vi "RT test - Copy.vi"() -> ()   [LabVIEW 2014]
uses:
  <vilib>/Platform/TimedLoop/XDataNode/timing_clust.ctl
  <vilib>/Platform/TimedLoop/XDataNode/nitl_modes.ctl
  <vilib>/Platform/TimedLoop/XDataNode/wakeup.ctl
  <vilib>/FPGAPlugInAG/cRIO-9066/niLvFpga_Open_cRIO-9066.vi
  <vilib>/rvi/interface/common/dynamic/niFpgaDynamicAddResources.vi
  <vilib>/Utility/error.llb/Error Cluster From Error Code.vi
  <vilib>/rvi/errors/niLvFpgaAdjustHostInterfaceError.vi
  <vilib>/platform/TimedLoop/XDataNode/XDataNode.xnode
  <vilib>/rvi/interface/nirviOpenFPGA/nirviOpenFPGA.xnode
  FPGA Bitfiles/SMSLDrill_FPGATarget_SMSL-DrillFPGA_76AJMwWUk6w.lvbitx
  FPGA/SMSL-Drill FPGA.vi
  <vilib>/rvi/interface/nirviReadWriteControl/nirviReadWriteControl.xnode
  <vilib>/Platform/TimedLoop/XDataNode/XDNodeRunTimeDep.lvlib
  NiFpgaLv.dll
  <vilib>/rvi/interface/Simulation/niFpgaSimulationCallBeginRW.vi
  <vilib>/NI_Real-Time Target Support.lvlib
panel:
  in  "Enable/Disable":bool
  in  "Speed Command [Inch/S]":dbl
  in  "Inch / Step":dbl=0.1
  in  "Manual":bool
  in  "Frequency [Hz]":dbl
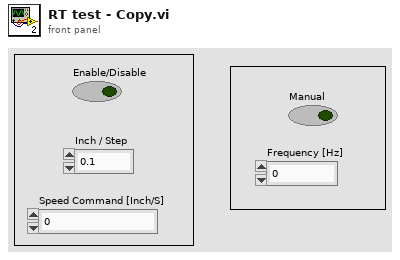
[diagram p1: front panel]
types:
  T1 = typedef "XDNodeRunTimeDep.lvlib/timing_clust.ctl" = cluster{"Expected End [f-1]":u64, "Actual End [f-1]":u64, "Finished Late? [f-1]":bool, "Expected End [i-1]":u64, "Actual End [i-1]":u64, "Finished Late? [i-1]":bool, "Expected Start [i]":u64, "Actual Start [i]":u64, "Expected Start [f]":u64, "Actual Start [f]":u64, "Source Name":string, "Structure Name":string, "Period":i64, "Deadline":i64, "Offset":i64, "Start":i64, "Priority":i32, "Timeout":i32, "Mode":T2, "Wakeup Reason":T3, "Error":errorcluster, "Source Type":string, "Secondary Source Type":string, "Global End Time":u64, "Global Start Time":u64, "Frame Duration":u64, "Iteration Duration":u64, "Assigned CPU":i32, "I/O Scan Engine Mode":u32}
  T2 = typedef "XDNodeRunTimeDep.lvlib/nitl_modes.ctl" = enum32{"No Change", "Process missed periods, maintain original phase", "Discard missed periods, maintain original phase", "Process missed periods, ignore original phase", "Discard missed periods, ignore original phase"}
  T3 = typedef "XDNodeRunTimeDep.lvlib/wakeup.ctl" = enum32{"Normal", "Aborted", "Asynchronous wakeup", "Timing source error", "Timed loop error", "Timeout"}
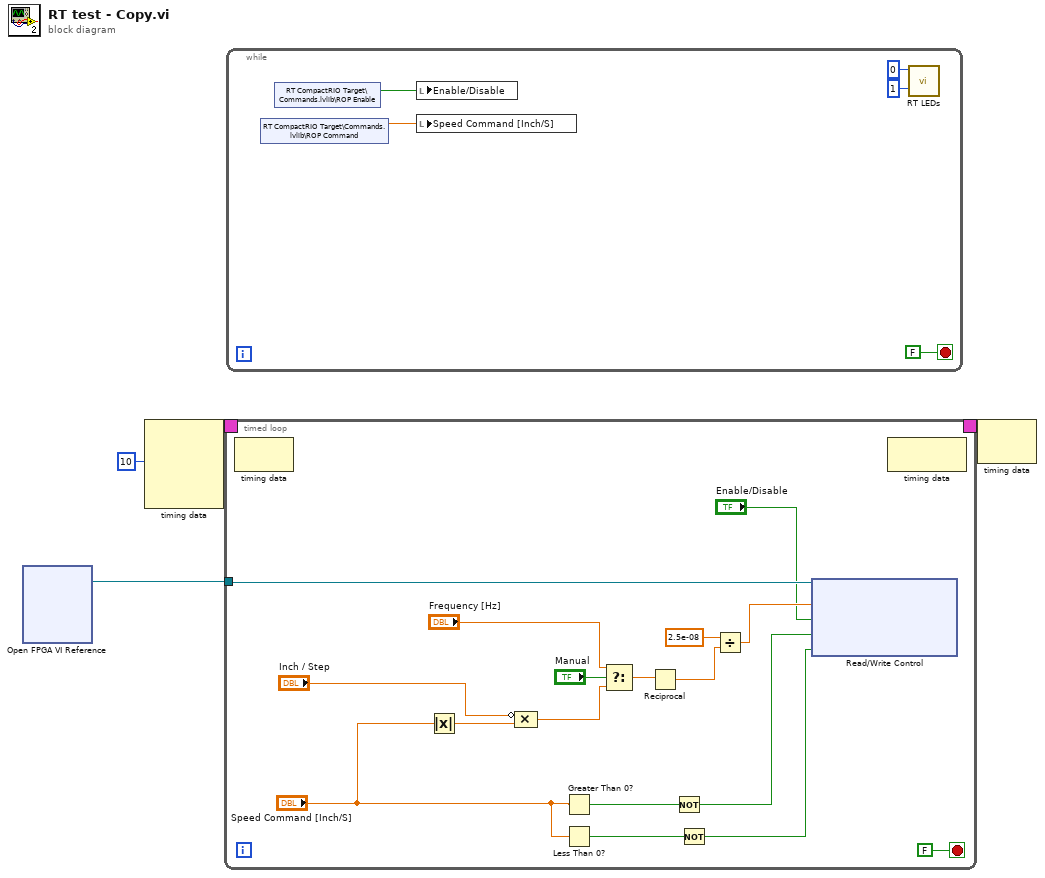
[diagram p0: block diagram]
diagram:
  n1 = xnode "Open FPGA VI Reference"() -> ("FPGA VI Reference Out"=w2:refnum<k20>)  [unwired: 2 in, 1 out]
  n2 = node-c288(i64 10 ("Period")) -> (w4:T1)  [unwired: 3 in]
  n3 = timed-loop {
    timing: w4 -> [_]
    timing-out: [_] -> w3
    tunnel: w2 -> [w21]
    stop <- FALSE stop-if-true
    n4 = node-c288() -> ()  [unwired: 1 in, 1 out]
    n5 = Absolute Value(x="Speed Command [Inch/S]") -> (abs(x)=w9:dbl)
    n6 = Compound Arithmetic op=MULTIPLY(invert "Inch / Step", w9) -> (w14:dbl)
    n7 = Greater Than 0?(x="Speed Command [Inch/S]") -> (x > 0?=w10:bool)
    n8 = Less Than 0?(x="Speed Command [Inch/S]") -> (x < 0?=w7:bool)
    n9 = Select(t="Frequency [Hz]", s="Manual", f=w14) -> (s? t:f=w17:dbl)
    n10 = Reciprocal(x=w17) -> (1/x=w18:dbl)
    n11 = Not(x=w10) -> (.not. x?=w6:bool)
    n12 = Not(x=w7) -> (.not. x?=w5:bool)
    n13 = Divide(x=2.5e-08 ("y"), y=w18) -> (x/y=w19:dbl)
    n14 = xnode "Read/Write Control"("FPGA VI Reference In"=w21, "frequency (periods/tick)"=w19, "Enable/Disable"="Enable/Disable", "Direction FWD"=w6, "Direction BKWD"=w5) -> ()  [unwired: 1 in, 2 out]
    n15 = node-c288() -> ()  [unwired: 1 in, 1 out]
  }
  n16 = while {
    stop <- FALSE stop-if-true
    n17 = shared-variable "RT CompactRIO Target\\Commands.lvlib\\ROP Command"() -> (w26:dbl)  [unwired: 1 in, 1 out]
    n18 = shared-variable "RT CompactRIO Target\\Commands.lvlib\\ROP Enable"() -> (w27:bool)  [unwired: 1 in, 1 out]
    n19 = local write "Enable/Disable"(w27) -> ()
    n20 = local write "Speed Command [Inch/S]"(w26) -> ()
    n21 = call <vilib>:"RT LEDs.vi"("State"=1, "LED Num"=0) -> ()  [unwired: 4 in, 2 out]
  }
  n22 = node-c288(w3) -> ()  [unwired: 1 out]
